vi "OpenOphir.vi"(0 "filter (0=out)":i32, 5 "wavelength":i32=2, 7 "range (0=auto)":i32, 11 "error in (no error)":errorcluster) -> (4 "OphirPM":T1={"Ophir-Ref"=refnum, "Ophir-Device"=1001, "Ophir-Channel"=0}, 15 "error out":errorcluster)   [LabVIEW 2012]
panel:
  out "Wavelength":string="828"
  out "Range":string="AUTO"
  out "Filter":string="OUT"
  out "serial #":string="538069"
  in  "OphirLMMeasurementLib.ICoLMMeasurement":refnum<k7> caption="OphirRefIn"
  # "OPHIR USBI Interface"
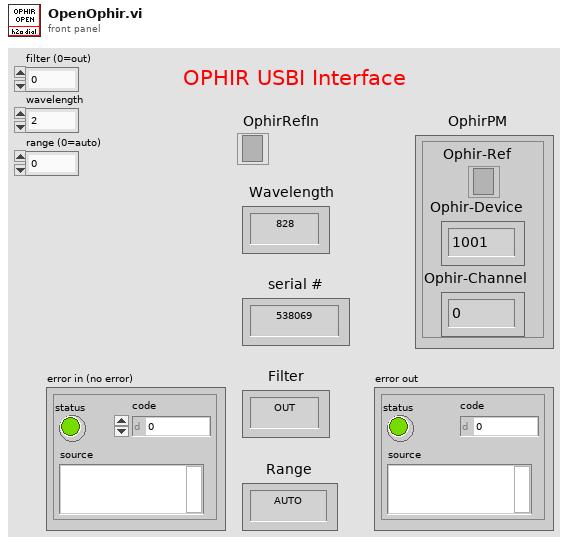
[diagram p1: front panel]
types:
  T1 = cluster{"Ophir-Ref":refnum<k7>, "Ophir-Device":i32, "Ophir-Channel":i32}
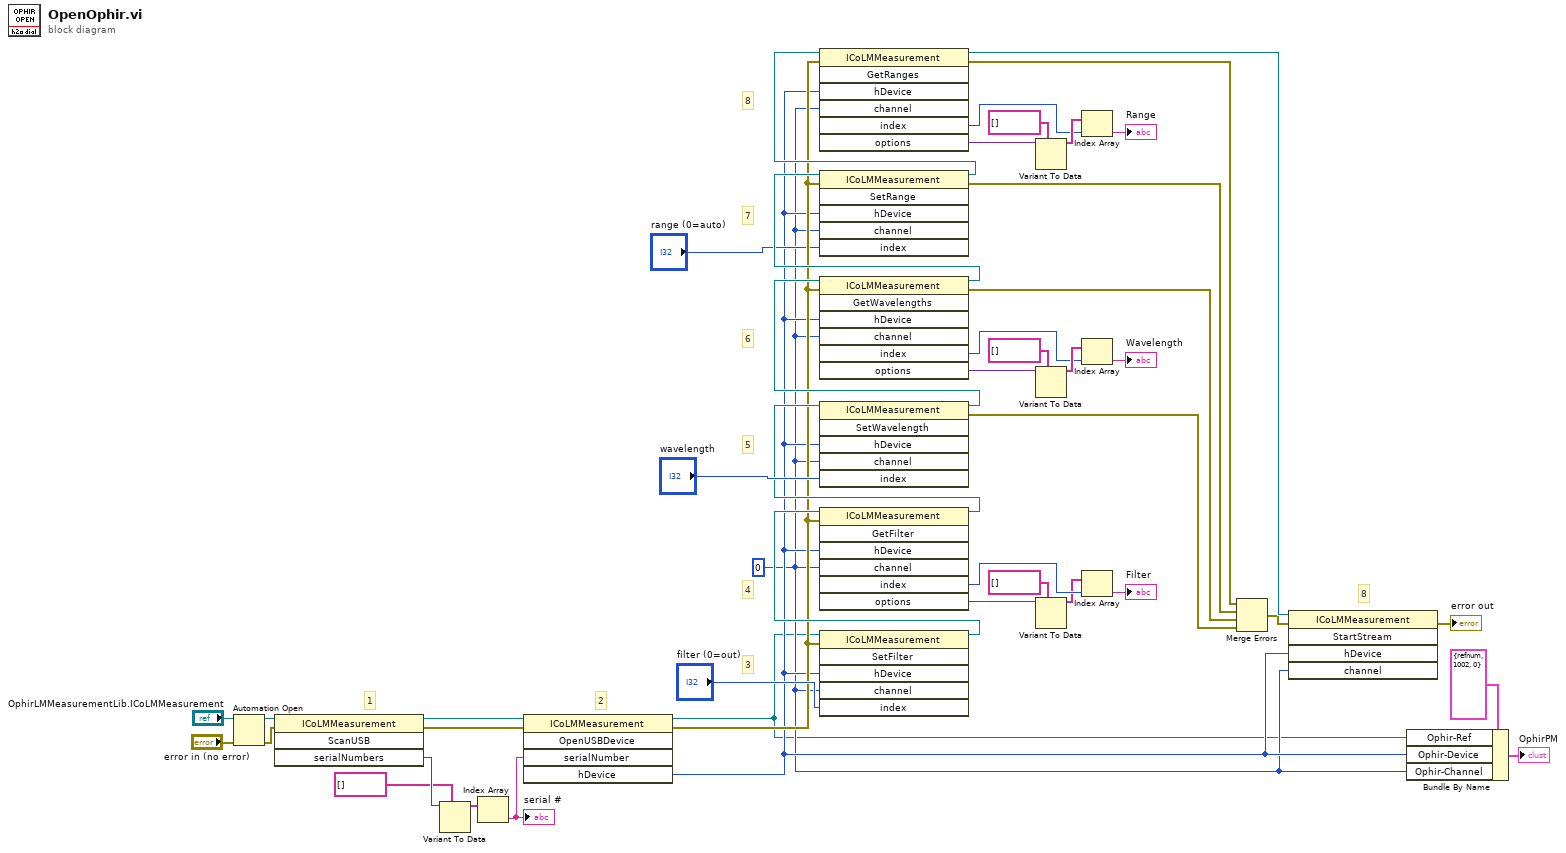
[diagram p0: block diagram]
diagram:
  w3 = 0 ("channel")
  # "8"
  # "8"
  # "7"
  # "6"
  # "5"
  # "4"
  # "3"
  # "2"
  # "1"
  n1 = Automation Open(error in (no error)="error in (no error)", Automation Refnum="OphirLMMeasurementLib.ICoLMMeasurement") -> (Automation Refnum=w45:refnum<k7>, error out=w39:errorcluster)  [unwired: 2 in]
  n2 = invoke class="ICoLMMeasurement" method="ScanUSB"(reference=w45, error in=w39) -> (reference out=w42:refnum<k7>, error out=w38:errorcluster, "serialNumbers"=w44:variant)  [unwired: 2 in, 1 out]
  n3 = Variant To Data(type=string[] [], Variant=w44) -> (data=w41:string[])  [unwired: 1 in, 1 out]
  n4 = Index Array(array=w41) -> (element=w40:string)  [unwired: 1 in]
  "serial #" <- w40
  n5 = invoke class="ICoLMMeasurement" method="OpenUSBDevice"(reference=w42, error in=w38, "serialNumber"=w40) -> (reference out=w1:refnum<k7>, error out=w9:errorcluster, "hDevice"=w4:i32)  [unwired: 2 in, 2 out]
  n6 = invoke class="ICoLMMeasurement" method="SetFilter"(reference=w1, error in=w9, "hDevice"=w4, "channel"=w3, "index"="filter (0=out)") -> (reference out=w36:refnum<k7>)  [unwired: 1 in, 5 out]
  n7 = invoke class="ICoLMMeasurement" method="GetFilter"(reference=w36, error in=w9, "hDevice"=w4, "channel"=w3) -> (reference out=w21:refnum<k7>, "index"=w30:i32, "options"=w35:variant)  [unwired: 3 in, 4 out]
  n8 = invoke class="ICoLMMeasurement" method="SetWavelength"(reference=w21, "hDevice"=w4, "channel"=w3, "index"="wavelength") -> (reference out=w20:refnum<k7>, error out=w16:errorcluster)  [unwired: 2 in, 4 out]
  n9 = invoke class="ICoLMMeasurement" method="GetWavelengths"(reference=w20, error in=w9, "hDevice"=w4, "channel"=w3) -> (reference out=w11:refnum<k7>, error out=w8:errorcluster, "index"=w18:i32, "options"=w33:variant)  [unwired: 3 in, 3 out]
  n10 = invoke class="ICoLMMeasurement" method="SetRange"(reference=w11, error in=w9, "hDevice"=w4, "channel"=w3, "index"="range (0=auto)") -> (reference out=w10:refnum<k7>, error out=w7:errorcluster)  [unwired: 1 in, 4 out]
  n11 = invoke class="ICoLMMeasurement" method="GetRanges"(reference=w10, error in=w9, "hDevice"=w4, "channel"=w3) -> (reference out=w15:refnum<k7>, error out=w23:errorcluster, "index"=w26:i32, "options"=w31:variant)  [unwired: 3 in, 3 out]
  n12 = Variant To Data(type=string[] [], Variant=w31) -> (data=w27:string[])  [unwired: 1 in, 1 out]
  n13 = Variant To Data(type=string[] [], Variant=w33) -> (data=w19:string[])  [unwired: 1 in, 1 out]
  n14 = Variant To Data(type=string[] [], Variant=w35) -> (data=w25:string[])  [unwired: 1 in, 1 out]
  n15 = Index Array(array=w27, index=w26) -> (element=→"Range":string)
  n16 = Index Array(array=w19, index=w18) -> (element=→"Wavelength":string)
  n17 = Index Array(array=w25, index=w30) -> (element=→"Filter":string)
  n18 = Merge Errors(w23, w7, w8, w16) -> (w14:errorcluster)
  n19 = invoke class="ICoLMMeasurement" method="StartStream"(reference=w15, error in=w14, "hDevice"=w4, "channel"=w3) -> (error out=→"error out":errorcluster)  [unwired: 1 in, 4 out]
  n20 = Bundle By Name(cluster=T1 {"Ophir-Ref"=refnum, "Ophir-Device"=1002, "Ophir-Channel"=0} ("OphirPM"), "Ophir-Ref"=w1, "Ophir-Device"=w4, "Ophir-Channel"=w3) -> (→"OphirPM":T1)
